vi "init.vi"(8 "error in":errorcluster, 10 "TBM module configuration in":refnum<class "TBM module configuration.lvclass">, 11 "testmod runtime in":refnum<class "testmod runtime.lvclass">) -> (0 "error out":errorcluster, 1 "data allocations":T1, 2 "execution settings":T4, 3 "testmod runtime out":refnum<class "testmod runtime.lvclass">)   [LabVIEW 2013, in "testmod runtime.lvclass"]
doc: "Provides an interface for initializing a module at runtime. While this interface performs no operations, a child should provide an override which may open any necessary references or sessions, allocate necessary memory, and perform any final configuration validataion before providing the full configuration <b>execution data</b> to the calling process."
uses:
  testmod runtime.lvclass
  <vilib>/NI/Tag Bus Module Framework/module configuration/TBM module configuration.lvclass
  <vilib>/NI/Tag Bus Module Framework/runtime/execution settings.ctl
  <vilib>/NI/Tag Bus Module Framework/channel/data tables.ctl
  <vilib>/NI/Tag Bus/dictionary/data dictionary.lvclass
  <vilib>/NI/Tag Bus/dictionary table pair.ctl
  <vilib>/NI/Tag Bus/table/data table.ctl
  configuration/testmod configuration.lvclass
  testmod runtime.lvclass/testmod runtime.ctl
  <vilib>/NI/Tag Bus Module Framework/channel/TBM channel.lvclass
  <vilib>/NI/Tag Bus Module Framework/runtime/TBM module execution interface.lvclass
  <vilib>/NI/Tag Bus/tag bus.lvlib
  <vilib>/NI/Tag Bus/table/data table.lvlib
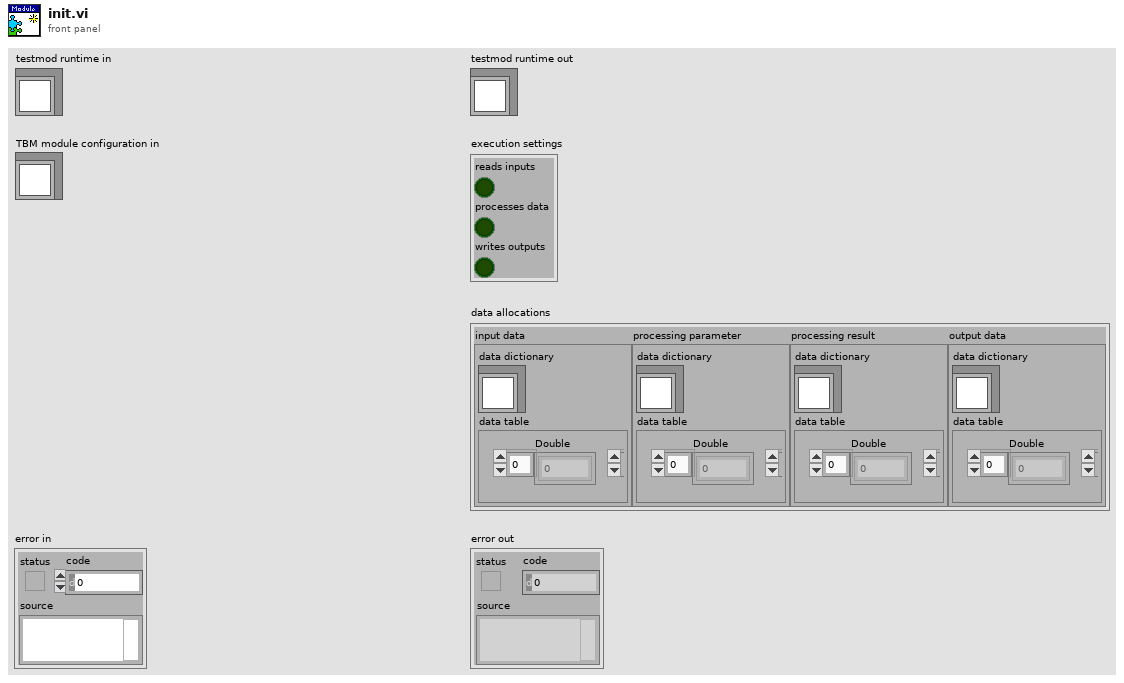
[diagram p1: front panel]
types:
  T1 = typedef "TBM channel.lvclass/data tables.ctl" = cluster{"input data":T2, "processing parameter":T2, "processing result":T2, "output data":T2}
  T2 = typedef "tag bus.lvlib/dictionary table pair.ctl" = cluster{"data dictionary":refnum<class "data dictionary.lvclass">, "data table":T3}
  T3 = typedef "tag bus.lvlib/data table.lvlib/data table.ctl" = cluster{"Double":dbl[], "Single":sgl[], "I64":i64[], "I32":i32[], "I16":i16[], "I8":i8[], "U64":u64[], "U32":u32[], "U16":u16[], "U8":u8[], "Boolean":bool[], "String":string[], "Array of Double":cluster{"DBL Array":dbl[]}[], "Array of Single":cluster{"SGL Array":sgl[]}[], "Array of I64":cluster{"I64 Array":i64[]}[], "Array of I32":cluster{"I32 Array":i32[]}[], "Array of I16":cluster{"I16 Array":i16[]}[], "Array of I8":cluster{"I8 Array":i8[]}[], "Array of U64":cluster{"U64 Array":u64[]}[], "Array of U32":cluster{"U32 Array":u32[]}[], "Array of U16":cluster{"U16 Array":u16[]}[], "Array of U8":cluster{"U8 Array":u8[]}[], "Array of Boolean":cluster{"Boolean Array":bool[]}[], "Array of String":cluster{"String Array":string[]}[]}
  T4 = typedef "TBM module execution interface.lvclass/execution settings.ctl" = cluster{"reads inputs":bool, "processes data":bool, "writes outputs":bool}
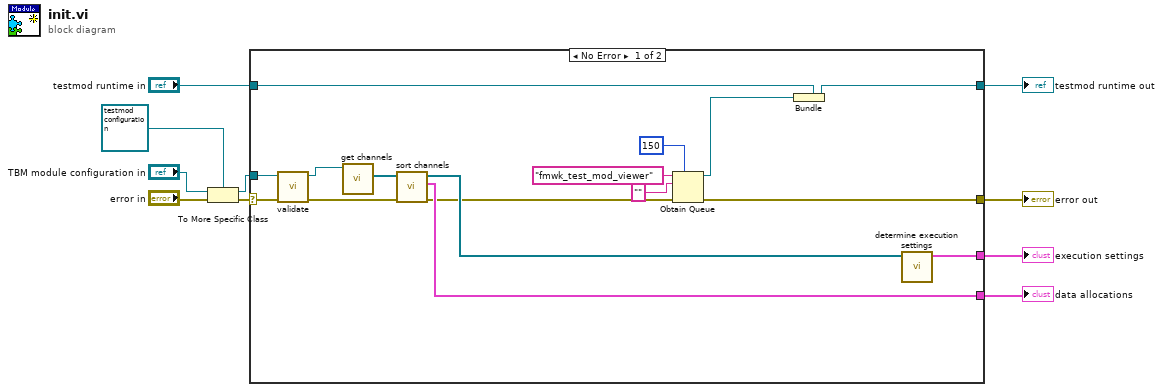
[diagram p0: block diagram]
diagram:
  n1 = To More Specific Class(target class=refnum<class "testmod configuration.lvclass"> refnum ("CVT configuration"), reference="TBM module configuration in", error in="error in") -> (specific class reference=w9:refnum<class "testmod configuration.lvclass">, error out=w10:errorcluster)
  n2 = case shown="No Error" w10 {
    selector: w10 -> [w22 w27]
    tunnel: w9 -> [w17 _]
    tunnel: "testmod runtime in" -> [w26 w28]
    tunnel: [w19 w28] -> w5
    tunnel: [w13 w27] -> w4
    tunnel: [w18 _] -> w2
    tunnel: [w25 _] -> w3
    frame No Error {
      n3 = call-dynamic "validate.vi"("error in"=w22, "CVT configuration in"=w17) -> ("error out"=w23:errorcluster, "CVT configuration out"=w21:refnum<class "testmod configuration.lvclass">)  [unwired: 8 in]
      n4 = call-dynamic "get channels.vi"("CVT configuration in"=w21) -> ("channels"=w20:refnum<class "TBM channel.lvclass">[])  [unwired: 9 in, 1 out]
      n5 = call <vilib>:"sort channels.vi"("error in"=w23, "channels in"=w20) -> ("error out"=w14:errorcluster, "data allocations"=w18:T1, "channels out"=w24:refnum<class "TBM channel.lvclass">[])  [unwired: 7 in]
      n6 = Obtain Queue(max queue size (-1, unlimited)=150, name (unnamed)="fmwk_test_mod_viewer", element data type="", error in (no error)=w14) -> (queue out=w12:refnum<queue>, error out=w13:errorcluster)  [unwired: 1 in, 1 out]
      n7 = Bundle(cluster=w26, w12) -> (w19:refnum<class "testmod runtime.lvclass">)
      n8 = call <vilib>:"determine execution settings.vi"("channels"=w24) -> ("execution settings"=w25:T4)  [unwired: 10 in]
    }
    frame Error {
    }
  }
  "error out" <- w4
  "testmod runtime out" <- w5
  "execution settings" <- w3
  "data allocations" <- w2
